vi "SaveFileBackGate.vi"(6 "DataIn":cluster{dbl[], "Ramp Pattern":dbl[]}, 8 "FileName":string, 10 "BG Time Taken (s)":dbl, 11 "Save To File":bool) -> ()   [LabVIEW 2019, in "SMU.lvclass"]
uses:
  SMU.lvclass
  <vilib>/Utility/file.llb/Write Delimited Spreadsheet (DBL).vi
  2231A/2231A.lvclass
panel:
  in  "File Name":string
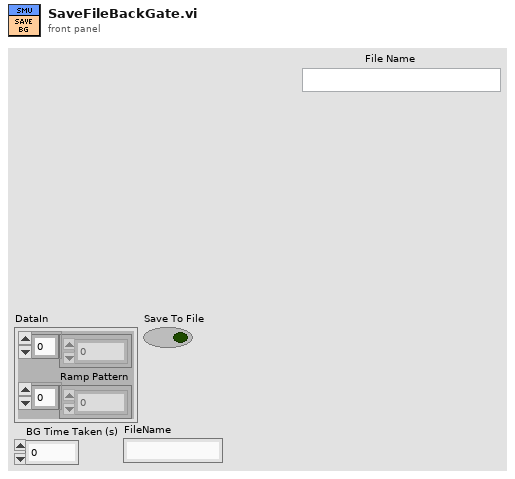
[diagram p1: front panel]
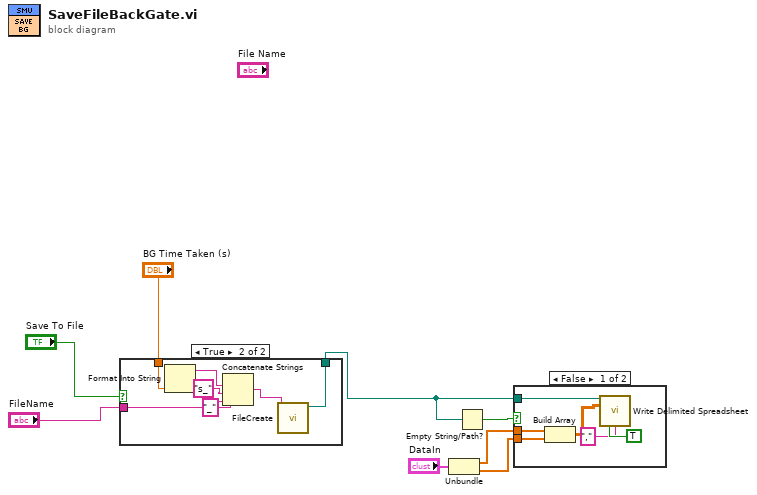
[diagram p0: block diagram]
diagram:
  n1 = case shown="True" "Save To File" {
    tunnel: "BG Time Taken (s)" -> [_ w15]
    tunnel: [_ w11] -> w1
    tunnel: "FileName" -> [_ w9]
    frame False {
    }
    frame True {
      n2 = Format Into String(w15) -> (resulting string=w14:string)  [unwired: 3 in, 1 out]
      n3 = Concatenate Strings("_" ("string"), w14, "s_" ("string"), w9) -> (w12:string)
      n4 = call "FileCreate.vi"("DAQ File Name"=w12) -> ("appended path 2"=w11:path)  [unwired: 9 in, 1 out]
    }
  }
  n5 = Unbundle("DataIn") -> (w7:dbl[], "Ramp Pattern"=w6:dbl[])
  n6 = Empty String/Path?(string/path=w1) -> (empty?=w2:bool)
  n7 = case shown="False" w2 {
    tunnel: w7 -> [w19 _]
    tunnel: w6 -> [w18 _]
    tunnel: w1 -> [w16 _]
    frame False {
      n8 = Build Array(w19, w18) -> (w17:dbl[][])
      n9 = call-poly <vilib>:"Write Delimited Spreadsheet.vi"("file path (dialog if empty)"=w16, "2D data"=w17, "transpose? (no:F)"=TRUE, "delimiter (\\t)"="," ("delimiter (\\t)")) -> ()  [unwired: 10 in, 2 out]
    }
    frame True {
    }
  }
